vi "Theta to X,Y.vi"(9 "theta":dbl, 10 "b":dbl, 11 "a":dbl) -> (3 "X,Y":dbl[](array[numeric]))   [LabVIEW 2021]
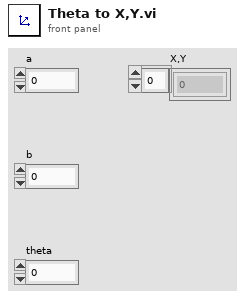
[diagram p1: front panel]
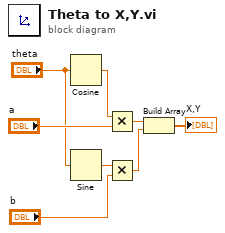
[diagram p0: block diagram]
diagram:
  n1 = Cosine(x="theta") -> (cos(x)=w2:dbl)
  n2 = Sine(x="theta") -> (sin(x)=w7:dbl)
  n3 = Multiply(x=w2, y="a") -> (x*y=w3:dbl)
  n4 = Multiply(x=w7, y="b") -> (x*y=w4:dbl)
  n5 = Build Array(w3, w4) -> (→"X,Y":dbl[])
